vi "record_async.vi"(3 "SSH password":string, 4 "Transfer and Run Date Folder After Experiment":bool, 5 "SSH user name":string, 6 "Tags":string, 7 "Frames":i32, 8 "Convert Power to Voltage":bool, 9 "voltages/power":dbl[](array[numeric]), 10 "parameters":string[](array[string]), 11 "parameters headers":string[](array[string])) -> ()   [LabVIEW 2016]
uses:
  <vilib>/vision/driver/IMAQdx.llb/IMAQdx Acquisition Mode.ctl
  <vilib>/userdefined/High Color/IMAQdx.ctl
  <vilib>/vision/driver/IMAQdx.llb/IMAQdx Buffer Number Mode.ctl
  <vilib>/Utility/file.llb/Write To Spreadsheet File (DBL).vi
  <vilib>/Utility/file.llb/Write To Spreadsheet File (string).vi
  <vilib>/Utility/file.llb/Read From Spreadsheet File (string).vi
  <vilib>/vision/driver/NI_Vision_Acquisition_Software.lvlib
panel:
  out "Saved Buffer Number":u32
  out "ProcessFrameRate":dbl
  out "# elements in queue":i32
  out "CameraFrameRate":dbl
  out "Camera Buffer Number":u32
  out "Image":T1(plugin-control)
  out "JPEG Quality":dbl
  out "Save Directory":path
  in  "stop":bool
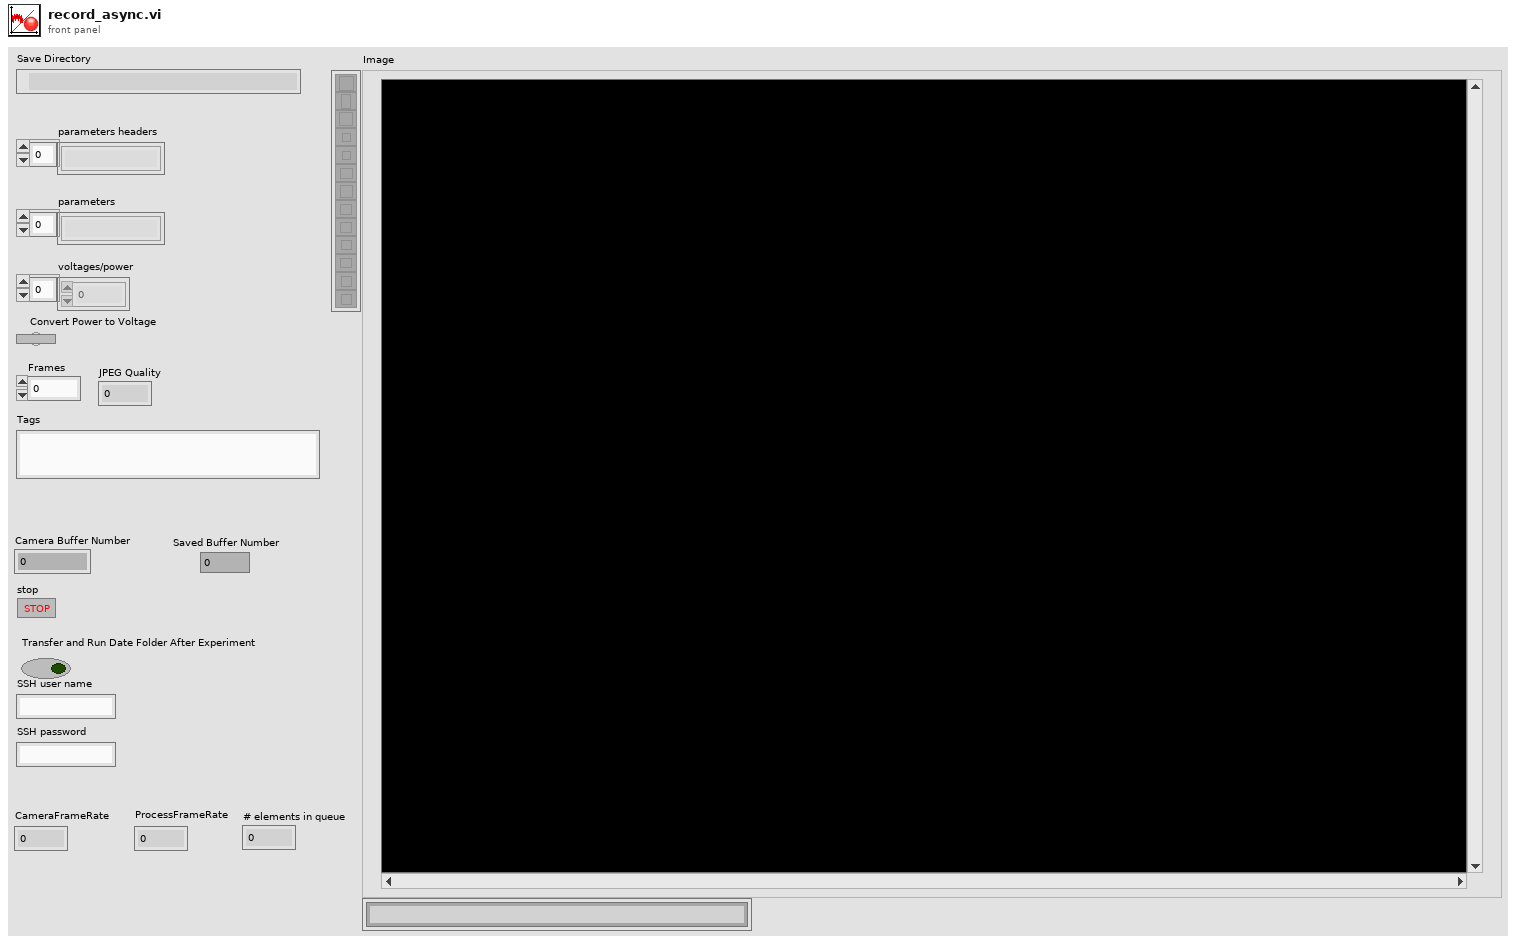
[diagram p1: front panel]
types:
  T1 = typedef "IMAQ Image.ctl" = refnum<image>
  T2 = typedef "IMAQdx.ctl" = refnum<k21>
  T3 = typedef "NI_Vision_Acquisition_Software.lvlib/IMAQdx Buffer Number Mode.ctl" = enum32{"Next", "Last", "Buffer Number", "Every", "Last New"}
  T4 = typedef "Image Type" = u32
  T5 = typedef "NI_Vision_Acquisition_Software.lvlib/IMAQdx Acquisition Mode.ctl" = enum32{"One Shot", "Continuous"}
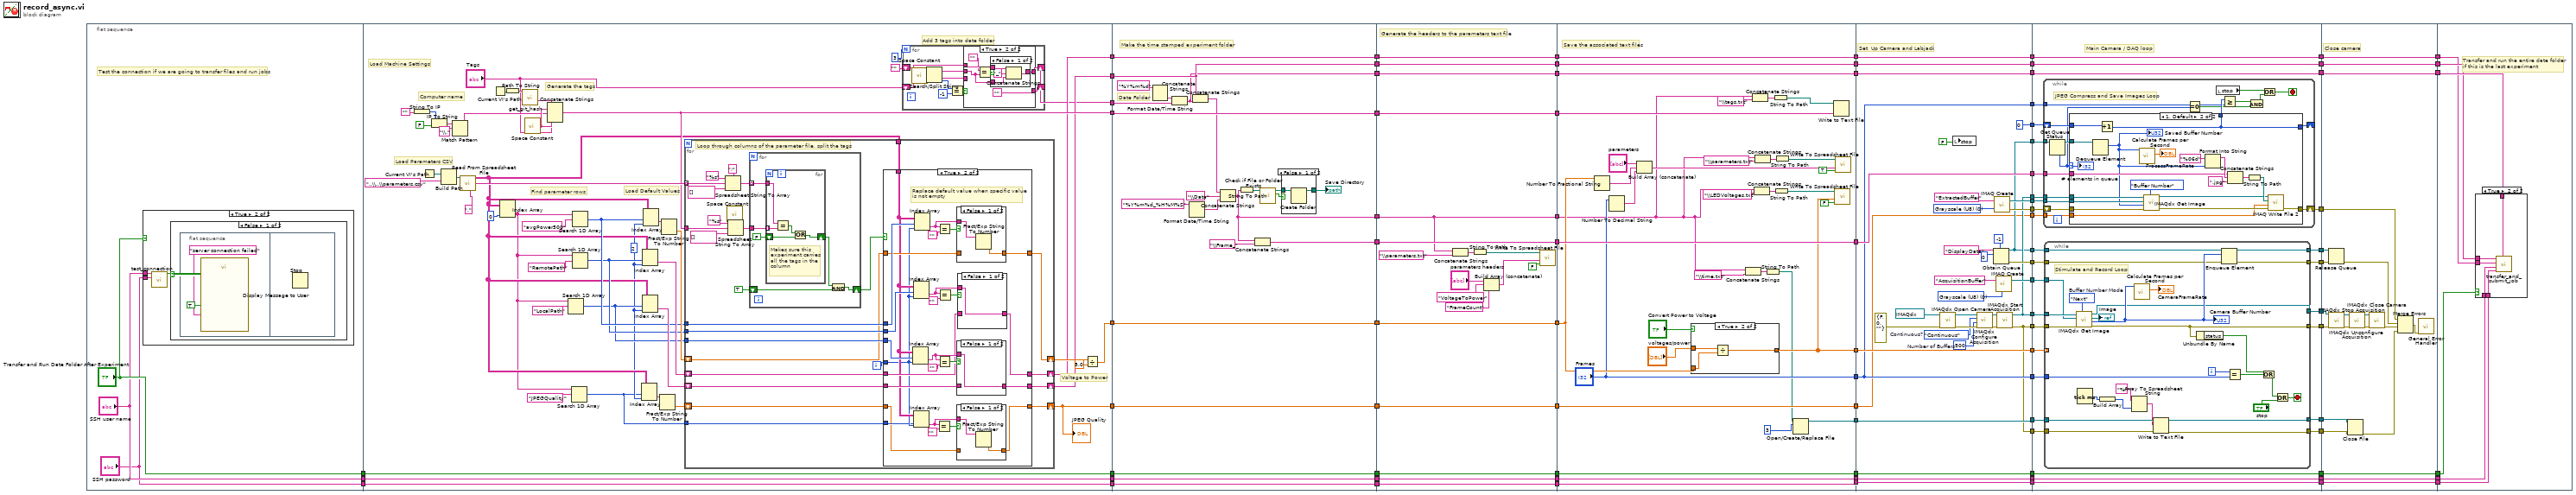
[diagram p0: block diagram]
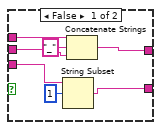
[diagram p4: hidden frame]
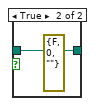
[diagram p11: hidden frame]
diagram:
  n1 = flat-sequence {
    tunnel: ["Transfer and Run Date Folder After Experiment"] -> w52
    tunnel: ["SSH user name"] -> w51
    tunnel: ["SSH password"] -> w50
    tunnel: [w134] -> w82
    tunnel: [w117] -> w81
    tunnel: [w108] -> w72
    tunnel: [w109] -> w71
    tunnel: w52 -> [w126]
    tunnel: w51 -> [w125]
    tunnel: w50 -> [w124]
    tunnel: [w126] -> w43
    tunnel: [w125] -> w36
    tunnel: [w124] -> w35
    tunnel: [w105] -> w28
    tunnel: [w96] -> w27
    tunnel: [w270] -> w66
    tunnel: [w269] -> w64
    tunnel: [w268] -> w62
    tunnel: [w267] -> w60
    tunnel: [w249] -> w58
    tunnel: [w251] -> w56
    tunnel: [w266] -> w54
    tunnel: w71 -> [w266]
    tunnel: w72 -> [w251]
    tunnel: w81 -> [w267]
    tunnel: w82 -> [w268]
    tunnel: [w258] -> w44
    tunnel: w43 -> [w258]
    tunnel: [w257] -> w37
    tunnel: w36 -> [w257]
    tunnel: w35 -> [w256]
    tunnel: [w256] -> w34
    tunnel: w28 -> [w252]
    tunnel: w27 -> [w248]
    tunnel: [w248] -> w24
    tunnel: w66 -> [w292]
    tunnel: [w292] -> w65
    tunnel: w64 -> [w278]
    tunnel: [w278] -> w63
    tunnel: w62 -> [w291]
    tunnel: [w291] -> w61
    tunnel: w60 -> [w290]
    tunnel: [w290] -> w59
    tunnel: w58 -> [w289]
    tunnel: [w289] -> w57
    tunnel: w56 -> [w288]
    tunnel: [w288] -> w55
    tunnel: w54 -> [w287]
    tunnel: [w287] -> w53
    tunnel: [w277] -> w45
    tunnel: w44 -> [w277]
    tunnel: [w276] -> w38
    tunnel: w37 -> [w276]
    tunnel: w34 -> [w275]
    tunnel: [w275] -> w33
    tunnel: [w274] -> w25
    tunnel: w24 -> [w274]
    tunnel: w65 -> [w325]
    tunnel: [w325] -> w87
    tunnel: [w309] -> w85
    tunnel: ["Frames"] -> w84
    tunnel: w63 -> [w296]
    tunnel: w61 -> [w305]
    tunnel: w59 -> [w300]
    tunnel: w57 -> [w314]
    tunnel: [w314] -> w77
    tunnel: [w313] -> w73
    tunnel: w55 -> [w313]
    tunnel: [w312] -> w67
    tunnel: w53 -> [w312]
    tunnel: [w303] -> w46
    tunnel: w45 -> [w303]
    tunnel: [w302] -> w39
    tunnel: w38 -> [w302]
    tunnel: w33 -> [w301]
    tunnel: [w301] -> w32
    tunnel: [w299] -> w26
    tunnel: w25 -> [w299]
    tunnel: [w294] -> w5
    tunnel: w87 -> [w339]
    tunnel: [w366] -> w86
    tunnel: w85 -> [w366]
    tunnel: w84 -> [w338]
    tunnel: [w338] -> w83
    tunnel: [w365] -> w78
    tunnel: w77 -> [w365]
    tunnel: [w364] -> w74
    tunnel: w73 -> [w364]
    tunnel: [w363] -> w68
    tunnel: w67 -> [w363]
    tunnel: [w362] -> w47
    tunnel: w46 -> [w362]
    tunnel: [w361] -> w40
    tunnel: w39 -> [w361]
    tunnel: w32 -> [w360]
    tunnel: [w360] -> w31
    tunnel: w26 -> [w336]
    tunnel: [w332] -> w23
    tunnel: [w340] -> w22
    tunnel: [w344] -> w21
    tunnel: [w343] -> w20
    tunnel: [w337] -> w19
    tunnel: [w342] -> w16
    tunnel: [w341] -> w15
    tunnel: [w340] -> w14
    tunnel: [w339] -> w13
    tunnel: [w338] -> w12
    tunnel: [w337] -> w11
    tunnel: [w336] -> w10
    tunnel: [0] -> w7
    tunnel: w5 -> [w333]
    tunnel: [w333] -> w4
    tunnel: [w332] -> w2
    tunnel: w86 -> [w396]
    tunnel: w83 -> [w395]
    tunnel: [w394] -> w79
    tunnel: w78 -> [w394]
    tunnel: [w393] -> w75
    tunnel: w74 -> [w393]
    tunnel: [w392] -> w69
    tunnel: w68 -> [w392]
    tunnel: [w391] -> w48
    tunnel: w47 -> [w391]
    tunnel: [w390] -> w41
    tunnel: w40 -> [w390]
    tunnel: w31 -> [w389]
    tunnel: [w389] -> w30
    tunnel: w23 -> [w388]
    tunnel: w22 -> [w387]
    tunnel: w21 -> [w386]
    tunnel: w20 -> [w385]
    tunnel: w19 -> [w384]
    tunnel: [w383] -> w18
    tunnel: [w382] -> w17
    tunnel: w16 -> [w381]
    tunnel: w15 -> [w380]
    tunnel: w14 -> [w379]
    tunnel: w13 -> [w378]
    tunnel: w12 -> [w377]
    tunnel: w11 -> [w376]
    tunnel: w10 -> [w375]
    tunnel: [w372] -> w9
    tunnel: [w374] -> w8
    tunnel: w7 -> [w373]
    tunnel: [w371] -> w6
    tunnel: w4 -> [w370]
    tunnel: [w369] -> w3
    tunnel: w2 -> [w368]
    tunnel: [w367] -> w1
    tunnel: [w484] -> w80
    tunnel: w79 -> [w484]
    tunnel: [w483] -> w76
    tunnel: w75 -> [w483]
    tunnel: [w482] -> w70
    tunnel: w69 -> [w482]
    tunnel: [w481] -> w49
    tunnel: w48 -> [w481]
    tunnel: [w480] -> w42
    tunnel: w41 -> [w480]
    tunnel: w30 -> [w479]
    tunnel: [w479] -> w29
    tunnel: w18 -> [w474]
    tunnel: w17 -> [w473]
    tunnel: w9 -> [w470]
    tunnel: w8 -> [w469]
    tunnel: w6 -> [w468]
    tunnel: w3 -> [w467]
    tunnel: w1 -> [w466]
    tunnel: w80 -> [w490]
    tunnel: w76 -> [w489]
    tunnel: w70 -> [w488]
    tunnel: w49 -> [w487]
    tunnel: w42 -> [w486]
    tunnel: w29 -> [w485]
    frame #0 {
      # "Test the connection if we are going to transfer files and run jobs"
      n2 = case shown="True" "Transfer and Run Date Folder After Experiment" {
        tunnel: "SSH password" -> [_ w93]
        tunnel: "SSH user name" -> [_ w91]
        frame False {
        }
        frame True {
          n3 = call "test_connection.vi"("Username"=w91, "Password"=w93) -> ("Connection Successful"=w92:bool)  [unwired: 7 in]
          n4 = case shown="False" w92 {
            frame False {
              n5 = flat-sequence {
                frame #0 {
                  n6 = call "Display Message to User"("Enable"=TRUE, "Message"="server connection failed") -> ()  [unwired: 8 in, 2 out]
                }
                frame #1 {
                  n7 = Stop() -> ()  [unwired: 1 in]
                }
              }
            }
            frame True {
            }
          }
        }
      }
    }
    frame #1 {
      w99 = 2
      # "Add 3 tags into date folder"
      # "Generate the tags"
      # "Find parameter rows"
      # "Load Default Values"
      # "Voltage to Power"
      # "Load Parameters CSV"
      # "Computer name"
      # "Load Machine Settings"
      n8 = String To IP(1:"") -> (0:w142:u32)
      n9 = Current VI's Path() -> (path=w137:path)
      n10 = IP To String(1:FALSE, 2:w142) -> (0:w139:string)
      n11 = Build Path(base path=w137, name or relative path="..\\..\\parameters.csv") -> (appended path=w128:path)
      n12 = Match Pattern(string=w139, regular expression="\\.") -> (before substring=w119:string)  [unwired: 1 in, 3 out]
      n13 = call-poly <vilib>:"Read From Spreadsheet File.vi"("delimiter (\\t)"=",", "file path (dialog if empty)"=w128) -> ("first row"=w118:string[], "all rows"=w101:string[][])  [unwired: 5 in, 3 out]
      n14 = Current VI's Path() -> (path=w121:path)
      n15 = Index Array(array=w101, index (col)=0) -> (element=w100:string[])  [unwired: 1 in]
      n16 = Path To String(path=w121) -> (string=w120:string)
      n17 = call "get_git_hash.vi"("VI folder"=w120) -> ("github hash"=w123:string)  [unwired: 10 in]
      n18 = call <vilib>:"Space Constant.vi"() -> ("String"=w122:string)
      n19 = Concatenate Strings(w123, w122, w119, w122, "Tags") -> (w117:string)
      n20 = Search 1D Array(1D array=w100, element="LocalPath") -> (index of element=w111:i32)  [unwired: 1 in]
      n21 = Search 1D Array(1D array=w100, element="JPEGQuality") -> (index of element=w97:i32)  [unwired: 1 in]
      n22 = Search 1D Array(1D array=w100, element="RemotePath") -> (index of element=w112:i32)  [unwired: 1 in]
      n23 = Search 1D Array(1D array=w100, element="avgPower500") -> (index of element=w113:i32)  [unwired: 1 in]
      n24 = Index Array(array=w101, index (row)=w97, index (col)=w99) -> (element=w102:string)
      n25 = Index Array(array=w101, index (row)=w112, index (col)=w99) -> (element=w115:string)
      n26 = Index Array(array=w101, index (row)=w111, index (col)=w99) -> (element=w114:string)
      n27 = Index Array(array=w101, index (row)=w113, index (col)=w99) -> (element=w130:string)
      n28 = Fract/Exp String To Number(string=w102) -> (number=w98:dbl)  [unwired: 3 in, 1 out]
      n29 = Fract/Exp String To Number(string=w130) -> (number=w116:dbl)  [unwired: 3 in, 1 out]
      n30 = for {
        tunnel: w118 -> [w196] mode=indexing
        tunnel: w117 -> [w188]
        tunnel: w113 -> [w183]
        tunnel: w112 -> [w182]
        tunnel: w111 -> [w181]
        tunnel: w101 -> [w186]
        shift-right: [w178] -> w110
        shift-left: w116 -> [w179]
        shift-right: [w175] -> w109
        shift-left: w115 -> [w176]
        shift-right: [w174] -> w108
        shift-left: w114 -> [w177]
        shift-right: [w171] -> w96
        shift-left: w98 -> [w173]
        tunnel: w97 -> [w172]
        i -> [w180]
        # "Loop through columns of the parameter file, split the tags"
        n31 = Spreadsheet String To Array(delimiter (Tab)=";", format string="%s", spreadsheet string=w196, array type (2D Dbl)=string[] []) -> (array=w192:string[])
        n32 = call <vilib>:"Space Constant.vi"() -> ("String"=w190:string)
        n33 = Spreadsheet String To Array(delimiter (Tab)=w190, format string="%s", spreadsheet string=w188, array type (2D Dbl)=string[] []) -> (array=w187:string[])
        n34 = for {
          tunnel: w192 -> [w242] mode=indexing
          tunnel: w187 -> [w241]
          shift-right: [w239] -> w184
          shift-left: TRUE -> [w237]
          n35 = for {
            tunnel: w242 -> [w247]
            tunnel: w241 -> [w246] mode=indexing
            shift-right: [w243] -> w238
            shift-left: FALSE -> [w244]
            # "Makes sure this\nexperiment carries\nall the tags in the\ncolumn"
            n36 = Equal?(x=w247, y=w246) -> (x = y?=w245:bool)
            n37 = Or(x=w245, y=w244) -> (x .or. y?=w243:bool)
          }
          n38 = And(x=w238, y=w237) -> (x .and. y?=w239:bool)
        }
        n39 = case shown="True" w184 {
          tunnel: w179 -> [w200 w221]
          tunnel: [w200 w220] -> w178
          tunnel: w183 -> [_ w226]
          tunnel: w182 -> [_ w225]
          tunnel: w181 -> [_ w224]
          tunnel: w180 -> [_ w203]
          tunnel: w186 -> [_ w204]
          tunnel: [w199 w210] -> w175
          tunnel: [w198 w212] -> w174
          tunnel: w177 -> [w198 w211]
          tunnel: w176 -> [w199 w209]
          tunnel: w173 -> [w197 w201]
          tunnel: w172 -> [_ w202]
          tunnel: [w197 w205] -> w171
          frame False {
          }
          frame True {
            # "Replace default value when specific value\nis not empty"
            n40 = Index Array(array=w204, index (row)=w224, index (col)=w203) -> (element=w213:string)
            n41 = Index Array(array=w204, index (row)=w225, index (col)=w203) -> (element=w216:string)
            n42 = Index Array(array=w204, index (row)=w202, index (col)=w203) -> (element=w206:string)
            n43 = Index Array(array=w204, index (row)=w226, index (col)=w203) -> (element=w219:string)
            n44 = Equal?(x=w206, y="") -> (x = y?=w207:bool)
            n45 = Equal?(x=w219, y="") -> (x = y?=w222:bool)
            n46 = Equal?(x=w213, y="") -> (x = y?=w214:bool)
            n47 = Equal?(x=w216, y="") -> (x = y?=w217:bool)
            n48 = case shown="False" w207 {
              tunnel: w201 -> [_ w229]
              tunnel: [w228 w229] -> w205
              tunnel: w206 -> [w227 _]
              frame False {
                n49 = Fract/Exp String To Number(string=w227) -> (number=w228:dbl)  [unwired: 3 in, 1 out]
              }
              frame True {
              }
            }
            n50 = case shown="False" w222 {
              tunnel: w221 -> [_ w236]
              tunnel: [w235 w236] -> w220
              tunnel: w219 -> [w234 _]
              frame False {
                n51 = Fract/Exp String To Number(string=w234) -> (number=w235:dbl)  [unwired: 3 in, 1 out]
              }
              frame True {
              }
            }
            n52 = case shown="False" w214 {
              tunnel: w213 -> [w230 _]
              tunnel: [w230 w231] -> w212
              tunnel: w211 -> [_ w231]
              frame False {
              }
              frame True {
              }
            }
            n53 = case shown="False" w217 {
              tunnel: w216 -> [w232 _]
              tunnel: [w232 w233] -> w210
              tunnel: w209 -> [_ w233]
              frame False {
              }
              frame True {
              }
            }
          }
        }
      }
      "JPEG Quality" <- w96
      n54 = for {
        N: 3 -> [_]
        shift-right: [w143] -> _
        shift-left: "Tags" -> [w152]
        shift-right: [w145] -> w105
        shift-left: "" -> [w150]
        n55 = call <vilib>:"Space Constant.vi"() -> ("String"=w151:string)
        n56 = Search/Split String(string=w152, search string/char (-)=w151) -> (substring before match=w149:string, match + rest of string=w148:string, offset of match=w147:i32)  [unwired: 1 in]
        n57 = Equal?(x=w147, y=-1) -> (x = y?=w144:bool)
        n58 = case shown="True" w144 {
          tunnel: w150 -> [w153 w163]
          tunnel: w149 -> [w154 w160]
          tunnel: w148 -> [w155 _]
          tunnel: [w157 ""] -> w143
          tunnel: [w156 w162] -> w145
          frame False {
            n59 = String Subset(string=w155, offset (0)=1) -> (substring=w157:string)  [unwired: 1 in]
            n60 = Concatenate Strings(w153, "_", w154) -> (w156:string)
          }
          frame True {
            n61 = Equal?(x="", y=w160) -> (x = y?=w164:bool)
            n62 = case shown="False" w164 {
              tunnel: w163 -> [w167 w170]
              tunnel: [w168 w170] -> w162
              tunnel: w160 -> [w166 _]
              frame False {
                n63 = Concatenate Strings(w167, "_", w166) -> (w168:string)
              }
              frame True {
              }
            }
          }
        }
      }
      n64 = Divide(x=w110, y=5.0) -> (x/y=w134:dbl)
    }
    frame #2 {
      # "Make the time stamped experiment folder"
      # "Date Folder"
      n65 = Format Date/Time String(time format string (%c)="%Y%m%d") -> (date/time string=w253:string)  [unwired: 2 in]
      n66 = Concatenate Strings(w253, w252) -> (w249:string)
      n67 = Format Date/Time String(time format string (%c)="%Y%m%d_%H%M%S") -> (date/time string=w255:string)  [unwired: 2 in]
      n68 = Concatenate Strings(w251, w249) -> (w250:string)
      n69 = Concatenate Strings(w250, "\\Data", w255) -> (w269:string)
      n70 = String To Path(string=w269) -> (path=w261:path)
      n71 = Concatenate Strings(w269, "\\Frame_") -> (w270:string)
      n72 = call <vilib>:"Check if File or Folder Exists.vi"("path"=w261) -> ("file or folder exists?"=w264:bool, "dup path"=w263:path)  [unwired: 8 in, 1 out]
      n73 = case shown="False" w264 {
        tunnel: [w271 w273] -> w260
        tunnel: w263 -> [w272 w273]
        frame False {
          n74 = Create Folder(path (use dialog)=w272) -> (created path=w271:path)  [unwired: 2 in, 2 out]
        }
        frame True {
          (unwired) errorcluster {"status"=FALSE, "code"=0, "source"=""} ("error out")
        }
      }
      "Save Directory" <- w260
    }
    frame #3 {
      # "Generate the headers to the parameters text file"
      n75 = Concatenate Strings(w278, "\\parameters.txt") -> (w286:string)
      n76 = String To Path(string=w286) -> (path=w285:path)
      n77 = Build Array (concatenate)("parameters headers", "VoltageToPower", "FrameCount") -> (w282:string[])
      n78 = call-poly <vilib>:"Write To Spreadsheet File.vi"("append to file? (new file:F)"=FALSE, "1D data"=w282, "file path (dialog if empty)"=w285) -> ()  [unwired: 5 in, 1 out]
    }
    frame #4 {
      # "Save the associated text files"
      n79 = Number To Fractional String(number=w305) -> (F-format string=w306:string)  [unwired: 3 in]
      n80 = Number To Decimal String(number="Frames") -> (decimal integer string=w307:string)  [unwired: 1 in]
      n81 = Build Array (concatenate)("parameters", w306, w307) -> (w318:string[])
      n82 = case shown="True" "Convert Power to Voltage" {
        tunnel: "voltages/power" -> [w328 w331]
        tunnel: [w328 w329] -> w309
        tunnel: w305 -> [_ w330]
        frame False {
        }
        frame True {
          n83 = Divide(x=w331, y=w330) -> (x/y=w329:dbl[])
        }
      }
      n84 = Concatenate Strings(w296, "\\time.txt") -> (w298:string)
      n85 = Concatenate Strings(w296, "\\tags.txt") -> (w316:string)
      n86 = Concatenate Strings(w296, "\\LEDVoltages.txt") -> (w327:string)
      n87 = Concatenate Strings(w296, "\\parameters.txt") -> (w322:string)
      n88 = String To Path(string=w298) -> (path=w295:path)
      n89 = String To Path(string=w316) -> (path=w315:path)
      n90 = String To Path(string=w327) -> (path=w326:path)
      n91 = String To Path(string=w322) -> (path=w321:path)
      n92 = Open/Create/Replace File(file path (use dialog)=w295, operation (0:open)=3) -> (refnum out=w294:refnum<file>)  [unwired: 4 in, 2 out]
      n93 = Write to Text File(file (use dialog)=w315, text=w300) -> ()  [unwired: 2 in, 3 out]
      n94 = call-poly <vilib>:"Write To Spreadsheet File.vi"("append to file? (new file:F)"=FALSE, "1D data"=w309, "file path (dialog if empty)"=w326) -> ()  [unwired: 5 in, 1 out]
      n95 = call-poly <vilib>:"Write To Spreadsheet File.vi"("append to file? (new file:F)"=TRUE, "1D data"=w318, "file path (dialog if empty)"=w321) -> ()  [unwired: 5 in, 1 out]
    }
    frame #5 {
      w347 = T4 0 items=["Grayscale (U8)", "Grayscale (I16)", "Grayscale (SGL)", "Complex (CSG)", "RGB (U32)", "HSL (U32)", "RGB (U64)"] ("Image Type")
      w356 = T4 0 items=["Grayscale (U8)", "Grayscale (I16)", "Grayscale (SGL)", "Complex (CSG)", "RGB (U32)", "HSL (U32)", "RGB (U64)"] ("Image Type")
      w357 = u32 500  # Number of Buffers
      w353 = IMAQdx_Acquisition_Mode."Continuous"  # Continuous?
      # "Set  Up Camera and Labjack"
      n96 = call <vilib>:"IMAQdx Open Camera.vi"("error in"=errorcluster {"status"=FALSE, "code"=0, "source"=""}, "Session In"=T2 "cam0") -> ("error out"=w358:errorcluster, "Session Out"=w359:T2)  [unwired: 8 in]
      n97 = local write "stop"(FALSE) -> ()
      n98 = call <vilib>:"IMAQdx Configure Acquisition.vi"("error in"=w358, "Number of Buffers"=w357, "Continuous?"=w353, "Session In"=w359) -> ("error out"=w354:errorcluster, "Session Out"=w352:T2)  [unwired: 6 in]
      n99 = Obtain Queue(max queue size (-1, unlimited)=-1, name (unnamed)="DisplayData", element data type=u32 0) -> (queue out=w337:refnum<queue>, error out=w343:errorcluster)  [unwired: 2 in, 1 out]
      n100 = call "IMAQ Create"("Image Name"="ExtractedBuffer", "Image Type"=w347) -> ("New Image"=w341:T1, "error out"=w342:errorcluster)  [unwired: 3 in]
      n101 = call "IMAQ Create"("Image Name"="AcquisitionBuffer", "Image Type"=w356) -> ("New Image"=w344:T1)  [unwired: 3 in, 1 out]
      n102 = call <vilib>:"IMAQdx Start Acquisition.vi"("error in"=w354, "Session In"=w352) -> ("error out"=w332:errorcluster, "Session Out"=w340:T2)  [unwired: 8 in]
    }
    frame #6 {
      # "Main Camera / DAQ loop"
      n103 = while {
        tunnel: w376 -> [w414]
        tunnel: w380 -> [w412]
        tunnel: w379 -> [w411]
        tunnel: w378 -> [w409]
        shift-right: [w408] -> w374
        shift-left: w381 -> [w410]
        tunnel: w377 -> [w401]
        tunnel: w375 -> [w406]
        shift-right: [w403] -> _
        shift-left: w373 -> [w404]
        stop <- w407 stop-if-true
        # "JPEG Compress and Save Images Loop"
        n104 = Get Queue Status(queue=w414) -> (queue out=w413:refnum<queue>, # elements in queue=w397:i32)  [unwired: 2 in, 6 out]
        n105 = case shown="1, Default" w397 {
          selector: w397 -> [_ w435]
          tunnel: w413 -> [_ w433]
          tunnel: w412 -> [_ w432]
          tunnel: w411 -> [_ w431]
          tunnel: w410 -> [w416 w430]
          tunnel: w409 -> [_ w424]
          tunnel: [w416 w420] -> w408
          tunnel: w406 -> [_ w419]
          tunnel: w404 -> [w415 w418]
          tunnel: [w415 w417] -> w403
          tunnel: [w415 w417] -> w402
          frame 0 {
          }
          frame 1, Default {
            n106 = Dequeue Element(queue=w433) -> (element=w421:u32)  [unwired: 2 in, 3 out]
            "Saved Buffer Number" <- w421
            n107 = Increment(x=w418) -> (x+1=w417:i32)
            n108 = call <vilib>:"Calculate Frames per Second.vi"("Buffer Number"=w421) -> ("Processed Frames/s"=→"ProcessFrameRate":dbl)  [unwired: 8 in, 2 out]
            n109 = call <vilib>:"IMAQdx Get Image.vi"("Buffer Number Mode (Next)"=IMAQdx_Buffer_Number_Mode."Buffer Number", "error in"=w430, "Buffer Number In"=w421, "Image In"=w432, "Session In"=w431) -> ("error out"=w422:errorcluster, "Image Out"=w423:T1)  [unwired: 3 in, 2 out]
            n110 = Format Into String(format string="%06d" ("string"), w421) -> (resulting string=w426:string)  [unwired: 2 in, 1 out]
            n111 = Concatenate Strings(w424, w426, ".jpg" ("string")) -> (w428:string)
            n112 = String To Path(string=w428) -> (path=w427:path)
            n113 = call-poly "IMAQ Write File 2"("error in (no error)"=w422, "Image Quality"=w419, "File Path"=w427, "Image"=w423) -> ("error out"=w420:errorcluster)  [unwired: 6 in, 1 out]
            "# elements in queue" <- w435
          }
        }
        n114 = Equal To 0?(x=w397) -> (x = 0?=w398:bool)
        n115 = local read "stop"() -> (w405:bool)
        n116 = Greater Or Equal?(x=w402, y=w401) -> (x >= y?=w400:bool)
        n117 = And(x=w400, y=w398) -> (x .and. y?=w399:bool)
        n118 = Or(x=w405, y=w399) -> (x .or. y?=w407:bool)
      }
      n119 = while {
        tunnel: w396 -> [_] mode=indexing
        tunnel: w395 -> [w461]
        tunnel: w388 -> [w456]
        tunnel: w387 -> [w455]
        tunnel: w386 -> [w454]
        tunnel: w385 -> [w453]
        tunnel: w384 -> [w452]
        tunnel: [w449] -> w371
        tunnel: [w448] -> w372
        tunnel: [w447] -> w383
        tunnel: [w446] -> w382
        tunnel: w370 -> [w444]
        tunnel: [w442] -> w369
        tunnel: w368 -> [w438]
        tunnel: [w437] -> w367
        i -> [w462]
        stop <- w464 stop-if-true
        w460 = IMAQdx_Buffer_Number_Mode."Next"  # Buffer Number Mode
        # "Stimulate and Record Loop"
        n120 = call <vilib>:"IMAQdx Get Image.vi"("Buffer Number Mode (Next)"=w460, "error in"=w456, "Image In"=w454, "Session In"=w455) -> ("error out"=w446:errorcluster, "Buffer Number Out"=w457:u32, "Image Out"=→"Image":T1, "Session Out"=w447:T2)  [unwired: 4 in]
        "Camera Buffer Number" <- w457
        n121 = Tick Count (ms)() -> (millisecond timer value=w441:u32)
        n122 = Build Array(w441) -> (w440:u32[])
        n123 = Array To Spreadsheet String(array=w440, 3:"%f") -> (spreadsheet string=w443:string)  [unwired: 1 in]
        n124 = call <vilib>:"Calculate Frames per Second.vi"("Buffer Number"=w457) -> ("Processed Frames/s"=→"CameraFrameRate":dbl)  [unwired: 8 in, 2 out]
        n125 = Write to Text File(file (use dialog)=w444, text=w443, error in=w438) -> (refnum out=w442:refnum<file>, error out=w437:errorcluster)  [unwired: 1 in, 1 out]
        n126 = Unbundle By Name(w446) -> ("status"=w451:bool)
        n127 = Enqueue Element(queue=w452, element=w457, error in (no error)=w453) -> (queue out=w449:refnum<queue>, error out=w448:errorcluster)  [unwired: 1 in, 1 out]
        n128 = Equal?(x=w462, y=w461) -> (x = y?=w445:bool)
        n129 = Or(x=w451, y=w445) -> (x .or. y?=w450:bool)
        n130 = Or(x=w450, y="stop") -> (x .or. y?=w464:bool)
      }
    }
    frame #7 {
      # "Close camera"
      n131 = Release Queue(queue=w468) -> ()  [unwired: 2 in, 3 out]
      n132 = call <vilib>:"IMAQdx Stop Acquisition.vi"("error in"=w473, "Session In"=w474) -> ("error out"=w475:errorcluster, "Session Out"=w476:T2)  [unwired: 8 in]
      n133 = Close File(refnum=w467, error in=w466) -> (error out=w465:errorcluster)  [unwired: 1 out]
      n134 = call <vilib>:"IMAQdx Unconfigure Acquisition.vi"("error in"=w475, "Session In"=w476) -> ("error out"=w478:errorcluster, "Session Out"=w477:T2)  [unwired: 8 in]
      n135 = call <vilib>:"IMAQdx Close Camera.vi"("error in"=w478, "Session In"=w477) -> ("error out"=w471:errorcluster)  [unwired: 9 in]
      n136 = Merge Errors(w469, w470, w471, w465) -> (w472:errorcluster)
      n137 = call <vilib>:"General Error Handler.vi"("error in (no error)"=w472) -> ()  [unwired: 10 in, 5 out]
    }
    frame #8 {
      # "Transfer and run the entire date folder\nif this is the last experiment"
      n138 = case shown="True" w487 {
        tunnel: w490 -> [_ w495]
        tunnel: w489 -> [_ w494]
        tunnel: w488 -> [_ w493]
        tunnel: w486 -> [_ w492]
        tunnel: w485 -> [_ w491]
        frame False {
        }
        frame True {
          n139 = call "transfer_and_submit_job.vi"("Date Folder"=w495, "Password"=w491, "Username"=w492, "Remote Data Directory"=w493, "Local Data Directory"=w494) -> ()  [unwired: 7 in]
        }
      }
    }
  }
